vi "Read sauce.vi"(8 "error in (no error)":errorcluster, 11 "Pizza":refnum<class "Pizza.lvclass">) -> (0 "error out":errorcluster, 2 "sauce":string, 3 "Pizza":refnum<class "Pizza.lvclass">)   [LabVIEW 2020, in "FactoryMethod.lvlib" / "PizzaFactoryMethod.lvlib" / "Pizza.lvclass"]
uses:
  Pizza.lvclass
  Pizza.lvclass/Pizza.ctl
  TypeDef/privateDataDVR.ctl
  TypeDef/privateData.ctl
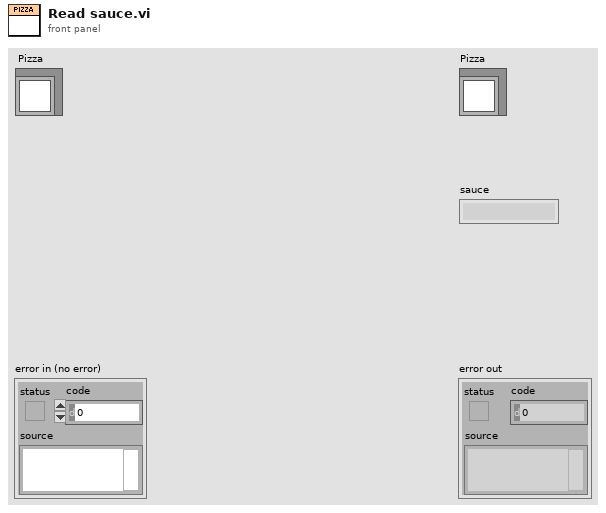
[diagram p1: front panel]
types:
  T1 = typedef "FactoryMethod.lvlib/PizzaFactoryMethod.lvlib/Pizza.lvclass/privateDataDVR.ctl" = refnum<data-value>
  T2 = typedef "FactoryMethod.lvlib/PizzaFactoryMethod.lvlib/Pizza.lvclass/privateData.ctl" = cluster{"name":string, "dough":string, "sauce":string, "toppings":string[]}
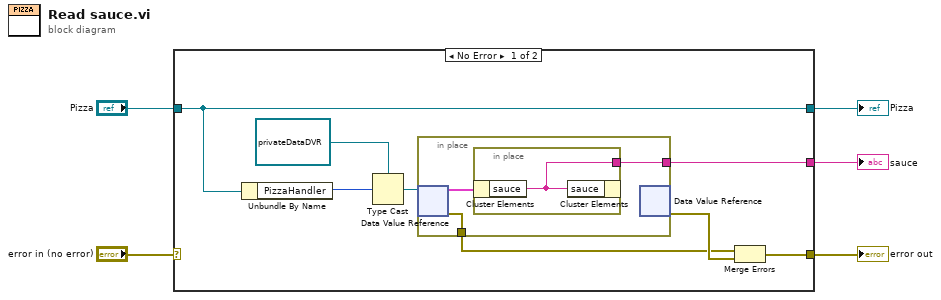
[diagram p0: block diagram]
diagram:
  n1 = case shown="No Error" "error in (no error)" {
    selector: "error in (no error)" -> [_ w19]
    tunnel: [w7 w19] -> w4
    tunnel: [w9 w18] -> w2
    tunnel: "Pizza" -> [w9 w18]
    tunnel: [w6 _] -> w1
    frame No Error {
      n2 = Unbundle By Name(w9) -> ("PizzaHandler"=w11:u32)
      n3 = Type Cast(type=T1 refnum ("privateDataDVR"), x=w11) -> (*(type *) &x=w13:T1)
      n4 = in-place {
        in-place-border: [w15] -> w6
        in-place-border: [w14] -> w10
        n5 = in-place-dvr #1(w13) -> (w16:T2, w14:errorcluster)
        n6 = in-place {
          in-place-border: [w17] -> w15
          n7 = in-place-cluster #2(w16) -> ("sauce"=w17:string)
          n8 = in-place-cluster #2("sauce"=w17) -> ()  [unwired: 1 out]
        }
        n9 = in-place-dvr #1() -> (w12:errorcluster)  [unwired: 1 in, 1 out]
      }
      n10 = Merge Errors(w10, w12) -> (w7:errorcluster)
    }
    frame Error {
    }
  }
  "error out" <- w4
  "Pizza" <- w2
  "sauce" <- w1
